vi "Scan Module.vi"(6 "Init":bool, 7 "Action":T1, 8 "Error In":errorcluster, 10 "Channel":u32(ring)=1 items=["A"=1, "B"=2, "A + B"=3, "C"=4, "A + C"=5, "A + B"=6, "D"=8, "A + D"=9, "B + D"=10, "C + D"=12, "A + B + C + D"=15], 11 "Mosaic Paramter":T2) -> (0 "Error Out":errorcluster, 1 "Current Position":cluster{"X":dbl, "Y":dbl}, 2 "Current State":T1, 3 "Finished?":bool)   [LabVIEW 2018]
uses:
  Controls/Go Scan Actions.ctl
  Controls/FGV Actions.ctl
  Hardware Mfg/Thorlabs Translation Stages/Controls/Motion Translation Module Control.ctl
  Hardware Mfg/Thorlabs Translation Stages/Controls/Translation Stage Cluster.ctl
  Controls/Translation Stage Types.ctl
  Controls/Set Get Controls.ctl
panel:
  out "Waveform Chart":dbl(graph)
  in  "No Slice?":bool
  out "XY Graph":cluster{"X":dbl, "Y":dbl}[](graph)
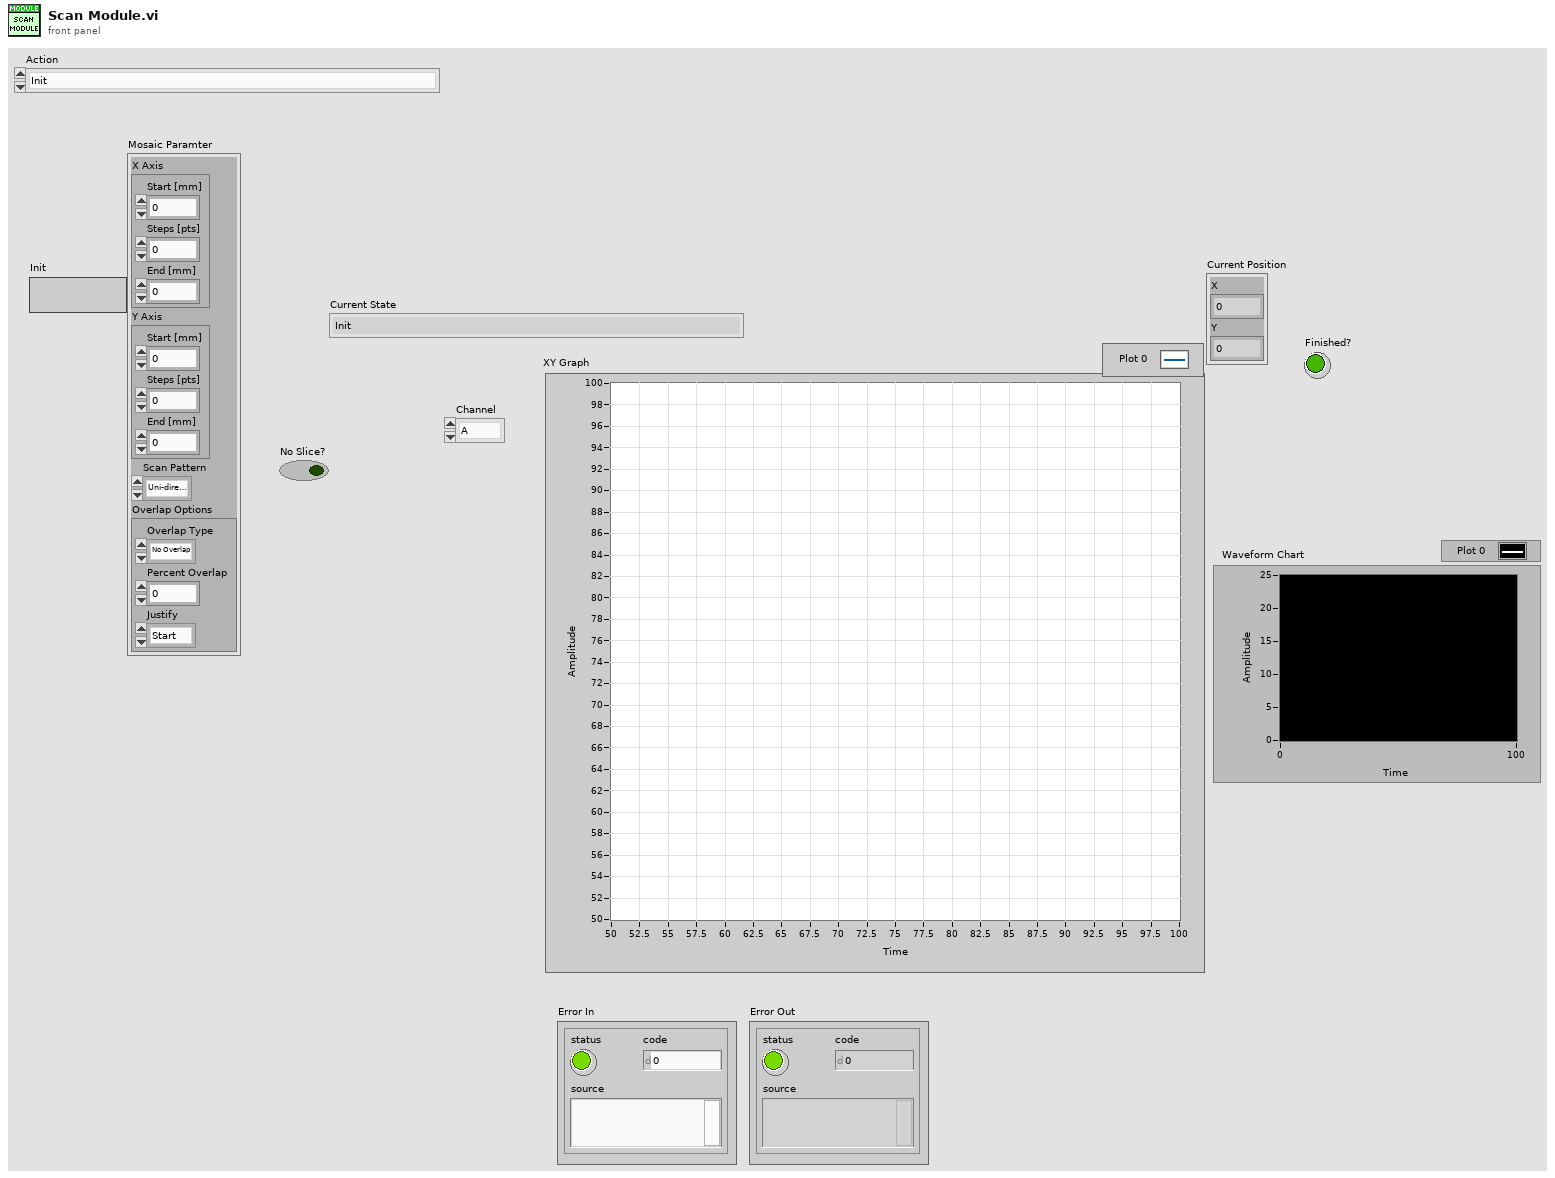
[diagram p1: front panel]
types:
  T1 = typedef "Go Scan Actions.ctl" = enum16{"Init", "Init Scan Head", "Init Table Stage", "Init Vibratome", "Generate Mosaic", "Go Image Home", "Go Mosaic", "Acquire Image", "Go Vibratome", "Slice", "Finished"}
  T2 = cluster{"X Axis":cluster{"Start [mm]":dbl, "Steps [pts]":u16, "End [mm]":dbl}, "Y Axis":cluster{"Start [mm]":dbl, "Steps [pts]":u16, "End [mm]":dbl}, "Scan Pattern":enum16{"Uni-directional", "Bi-Directional", "Spiral Out", "Spiral In"}, "Overlap Options":cluster{"Overlap Type":enum16{"No Overlap", "X Only", "Y Only", "X and Y"}, "Percent Overlap":u8, "Justify":enum16{"Start", "Center", "End"}}}
  T3 = typedef "FGV Actions.ctl" = enum16{"Init", "Set", "Get", "Clear"}
  T4 = typedef "Translation Stage Cluster.ctl" = cluster{"Position":dbl, "Is.Enabled?":bool, "Is.Connected?":bool, "Device SN":string, "AccelerationMaximum":dbl, "VelocityMaximum":dbl, "Acceleration":dbl, "Velocity":dbl, "waitTimeout (ms)":i32, "Model":T5, "Is.Homed?":bool}
  T5 = typedef "Translation Stage Types.ctl" = enum16{"None", "Thorlabs LTS", "Thorlabs MLJ"}
  T6 = typedef "Set Get Controls.ctl" = enum16{"Set", "Get"}
  T7 = typedef "Motion Translation Module Control.ctl" = enum16{"Init", "Home", "Status", "Velocity/Accel", "Position", "Jog", "Stop", "Uninit", "Enable", "Disable"}
  T8 = typedef "ScanType.ctl" = enum16{"Single Frame", "Continuous Frame", "ROI Line", "Vibratome", "Mosaic", "Mosaic + Slice"}
  T9 = cluster{"Start [mm]":dbl, "Steps [pts]":u16, "End [mm]":dbl}
  T10 = cluster{"Overlap Type":enum16{"No Overlap", "X Only", "Y Only", "X and Y"}, "Percent Overlap":u8, "Justify":enum16{"Start", "Center", "End"}}
  T11 = enum16{"Uni-directional", "Bi-Directional", "Spiral Out", "Spiral In"}
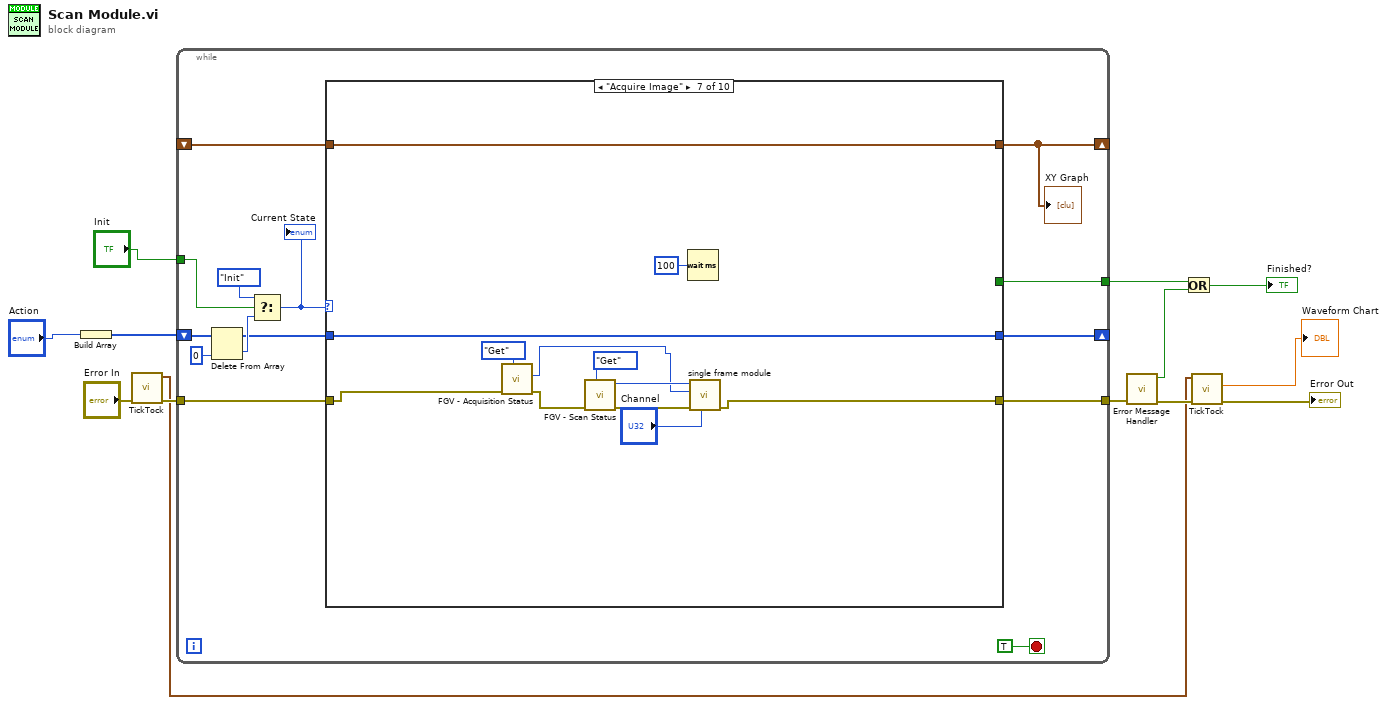
[diagram p0: block diagram]
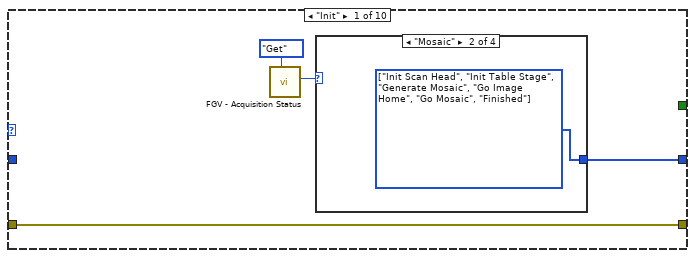
[diagram p2: hidden frame]
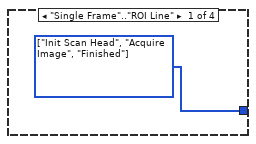
[diagram p3: hidden frame]
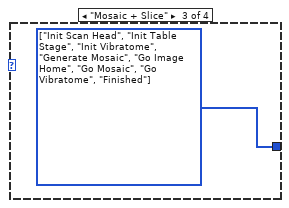
[diagram p4: hidden frame]
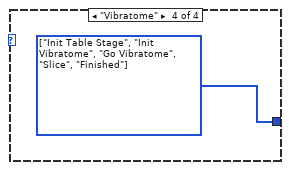
[diagram p5: hidden frame]
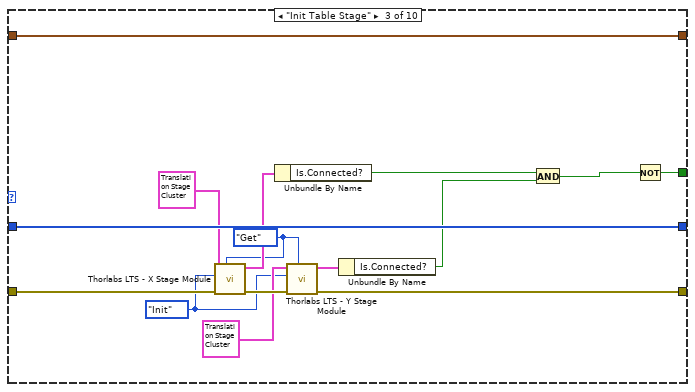
[diagram p7: hidden frame]
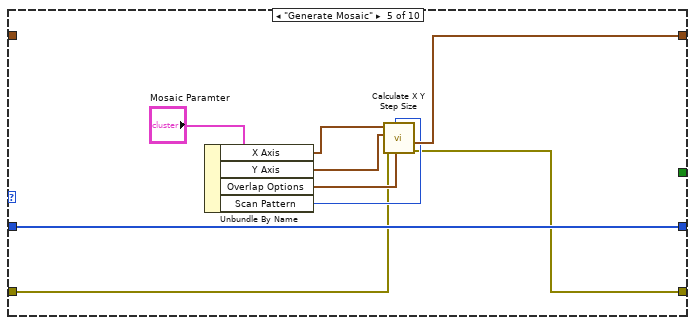
[diagram p9: hidden frame]
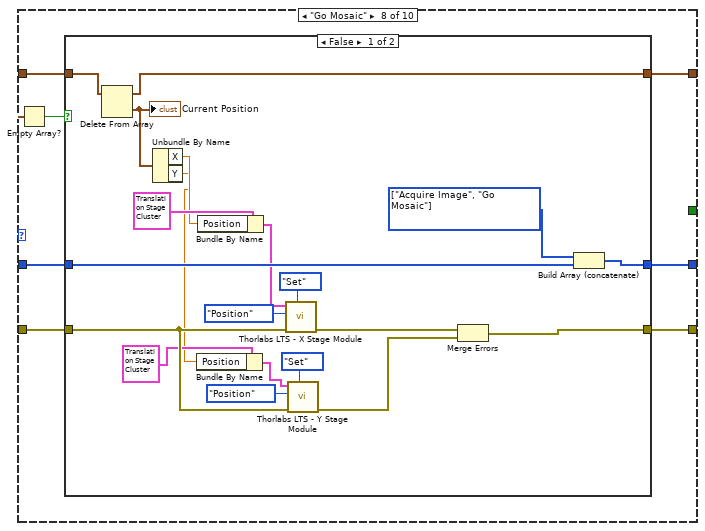
[diagram p11: hidden frame]
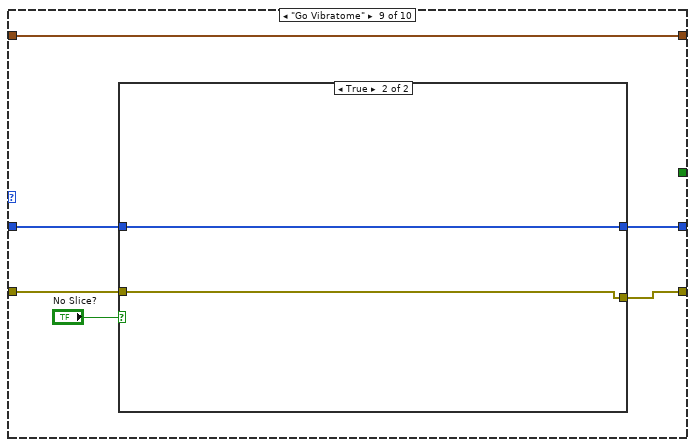
[diagram p13: hidden frame]
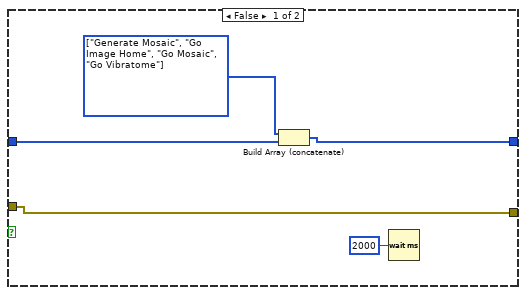
[diagram p14: hidden frame]
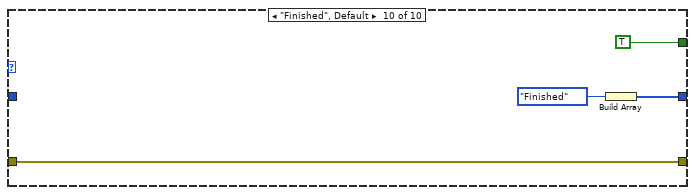
[diagram p15: hidden frame]
diagram:
  n1 = Build Array("Action") -> (w1:T1[])
  n2 = call "TickTock.vi"("Error In"="Error In") -> ("Error Out"=w6:errorcluster, "Current Time (Out)"=w4:timestamp)  [unwired: 8 in, 1 out]
  n3 = while {
    shift-right: [w23] -> _
    shift-left: w1 -> [w22]
    tunnel: "Init" -> [w25]
    shift-right: [w18] -> _
    shift-left: _ -> [w19]
    tunnel: [w17] -> w12
    tunnel: w6 -> [w15]
    tunnel: [w14] -> w11
    stop <- TRUE stop-if-true
    n4 = Delete From Array(array=w22, index=0) -> (deleted portion=w21:T1, array with subset deleted=w20:T1[])  [unwired: 1 in]
    n5 = Select(t=Go_Scan_Actions."Init", s=w25, f=w21) -> (s? t:f=w24:T1)
    "Current State" <- w24
    n6 = case shown="\"Acquire Image\"" w24 {
      tunnel: [w28 w37 w52 w55 w65 w67 w79 w83 w113 w126] -> w23
      tunnel: w20 -> [_ w37 w52 w55 w65 w67 w79 w84 w114 _]
      tunnel: [_ w38 w53 w56 w64 w68 w80 w87 w116 _] -> w18
      tunnel: w19 -> [_ w38 w53 w56 _ w68 w80 w86 w116 _]
      tunnel: [_ _ w47 _ _ _ _ _ _ TRUE] -> w17
      tunnel: w15 -> [w29 w36 w51 w54 w58 w66 w71 w82 w112 w124]
      tunnel: [w29 w36 w45 w54 w57 w66 w73 w81 w111 w124] -> w14
      frame "Init" {
        n7 = call "FGV - Acquisition Status.vi"("Actions"=FGV_Actions."Get") -> ("Scan Type [Out]"=w30:T8)  [unwired: 8 in, 2 out]
        n8 = case shown="\"Mosaic\"" w30 {
          tunnel: [w32 w33 w34 w35] -> w28
          frame "Single Frame".."ROI Line" {
            w32 = T1[] [enum."Init Scan Head", enum."Acquire Image", enum."Finished"] items=["Init", "Init Scan Head", "Init Table Stage", "Init Vibratome", "Generate Mosaic", "Go Image Home", "Go Mosaic", "Acquire Image", "Go Vibratome", "Slice", "Finished"]
          }
          frame "Mosaic" {
            w33 = T1[] [enum."Init Scan Head", enum."Init Table Stage", enum."Generate Mosaic", enum."Go Image Home", enum."Go Mosaic", enum."Finished"] items=["Init", "Init Scan Head", "Init Table Stage", "Init Vibratome", "Generate Mosaic", "Go Image Home", "Go Mosaic", "Acquire Image", "Go Vibratome", "Slice", "Finished"]
          }
          frame "Mosaic + Slice" {
            w34 = T1[] [enum."Init Scan Head", enum."Init Table Stage", enum."Init Vibratome", enum."Generate Mosaic", enum."Go Image Home", enum."Go Mosaic", enum."Go Vibratome", enum."Finished"] items=["Init", "Init Scan Head", "Init Table Stage", "Init Vibratome", "Generate Mosaic", "Go Image Home", "Go Mosaic", "Acquire Image", "Go Vibratome", "Slice", "Finished"]
          }
          frame "Vibratome" {
            w35 = T1[] [enum."Init Table Stage", enum."Init Vibratome", enum."Go Vibratome", enum."Slice", enum."Finished"] items=["Init", "Init Scan Head", "Init Table Stage", "Init Vibratome", "Generate Mosaic", "Go Image Home", "Go Mosaic", "Acquire Image", "Go Vibratome", "Slice", "Finished"]
          }
        }
      }
      frame "Init Scan Head" {
      }
      frame "Init Table Stage" {
        w39 = Set_Get_Controls."Get" ("Set/Get")
        w43 = Motion_Translation_Module_Control."Init" ("Action")
        n9 = call "Thorlabs LTS - X Stage Module.vi"("Set/Get"=w39, "Error In"=w51, "Action"=w43, "Cluster In"=T4 {"Position"=0.0, "Is.Enabled?"=TRUE, "Is.Connected?"=FALSE, "Device SN"="45876060", "AccelerationMaximum"=0.0, "VelocityMaximum"=0.0, "Acceleration"=0.0, "Velocity"=0.0, "waitTimeout (ms)"=10000, "Model"=enum."None", "Is.Homed?"=FALSE}) -> ("Error Out"=w50:errorcluster, "Cluster Out"=w49:T4)  [unwired: 6 in]
        n10 = Unbundle By Name(w49) -> ("Is.Connected?"=w48:bool)
        n11 = call "Thorlabs LTS - Y Stage Module.vi"("Set/Get"=w39, "Error In"=w50, "Action"=w43, "Cluster In"=T4 {"Position"=0.0, "Is.Enabled?"=TRUE, "Is.Connected?"=FALSE, "Device SN"="45876539", "AccelerationMaximum"=0.0, "VelocityMaximum"=0.0, "Acceleration"=0.0, "Velocity"=0.0, "waitTimeout (ms)"=10000, "Model"=enum."None", "Is.Homed?"=FALSE}) -> ("Error Out"=w45:errorcluster, "Cluster Out"=w42:T4)  [unwired: 6 in]
        n12 = Unbundle By Name(w42) -> ("Is.Connected?"=w40:bool)
        n13 = And(x=w48, y=w40) -> (x .and. y?=w41:bool)
        n14 = Not(x=w41) -> (.not. x?=w47:bool)
      }
      frame "Init Vibratome" {
      }
      frame "Generate Mosaic" {
        n15 = Unbundle By Name("Mosaic Paramter") -> ("X Axis"=w62:T9, "Y Axis"=w61:T9, "Overlap Options"=w60:T10, "Scan Pattern"=w59:T11)
        n16 = call "Calculate X Y Step Size.vi"("Overlap Options"=w60, "Scan Pattern"=w59, "Error In"=w58, "Y Axis"=w61, "X Axis"=w62) -> ("Error Out"=w57:errorcluster, "Array"=w64:cluster{"X":dbl, "Y":dbl}[])  [unwired: 3 in, 2 out]
      }
      frame "Go Image Home" {
      }
      frame "Acquire Image" {
        n17 = call "FGV - Acquisition Status.vi"("Actions"=FGV_Actions."Get", "Error In"=w71) -> ("Error Out"=w70:errorcluster, "Scan Type [Out]"=w69:T8)  [unwired: 7 in, 1 out]
        n18 = call "FGV - Scan Status.vi"("Actions"=FGV_Actions."Get", "Error In"=w70) -> ("Error Out"=w76:errorcluster, "Scan Status out"=w75:enum16{"Start", "Continue Scan", "Finish Scan"})  [unwired: 7 in, 1 out]
        n19 = Wait (ms)(milliseconds to wait=u32 100) -> ()  [unwired: 1 out]
        n20 = call "single frame module.vi"("Channel"="Channel", "Error in"=w76, "Scan Type in"=w69, "Scan Status in"=w75) -> ("Error Out"=w73:errorcluster)  [unwired: 7 in]
      }
      frame "Go Mosaic" {
        n21 = Empty Array?(array=w86) -> (empty?=w85:bool)
        n22 = case shown="False" w85 {
          tunnel: [w107 w110] -> w87
          tunnel: w86 -> [w106 w110]
          tunnel: w84 -> [w105 w109]
          tunnel: [w103 w109] -> w83
          tunnel: w82 -> [w93 w108]
          tunnel: [w89 w108] -> w81
          frame False {
            w102 = T1[] [enum."Acquire Image", enum."Go Mosaic"] items=["Init", "Init Scan Head", "Init Table Stage", "Init Vibratome", "Generate Mosaic", "Go Image Home", "Go Mosaic", "Acquire Image", "Go Vibratome", "Slice", "Finished"]
            n23 = Delete From Array(array=w106) -> (deleted portion=w104:cluster{"X":dbl, "Y":dbl}, array with subset deleted=w107:cluster{"X":dbl, "Y":dbl}[])  [unwired: 2 in]
            "Current Position" <- w104
            n24 = Unbundle By Name(w104) -> ("X"=w97:dbl, "Y"=w91:dbl)
            n25 = Bundle By Name(cluster=T4 {"Position"=0.0, "Is.Enabled?"=FALSE, "Is.Connected?"=FALSE, "Device SN"="45876539", "AccelerationMaximum"=0.0, "VelocityMaximum"=0.0, "Acceleration"=0.0, "Velocity"=0.0, "waitTimeout (ms)"=10000, "Model"=enum."None", "Is.Homed?"=FALSE} ("Cluster In"), "Position"=w91) -> (w90:T4)
            n26 = Bundle By Name(cluster=T4 {"Position"=0.0, "Is.Enabled?"=FALSE, "Is.Connected?"=FALSE, "Device SN"="45876539", "AccelerationMaximum"=0.0, "VelocityMaximum"=0.0, "Acceleration"=0.0, "Velocity"=0.0, "waitTimeout (ms)"=10000, "Model"=enum."None", "Is.Homed?"=FALSE} ("Cluster In"), "Position"=w97) -> (w96:T4)
            n27 = call "Thorlabs LTS - X Stage Module.vi"("Set/Get"=Set_Get_Controls."Set", "Error In"=w93, "Action"=Motion_Translation_Module_Control."Position", "Cluster In"=w96) -> ("Error Out"=w100:errorcluster)  [unwired: 6 in, 1 out]
            n28 = call "Thorlabs LTS - Y Stage Module.vi"("Set/Get"=Set_Get_Controls."Set", "Error In"=w93, "Action"=Motion_Translation_Module_Control."Position", "Cluster In"=w90) -> ("Error Out"=w88:errorcluster)  [unwired: 6 in, 1 out]
            n29 = Merge Errors(w100, w88) -> (w89:errorcluster)
            n30 = Build Array (concatenate)(w102, w105) -> (w103:T1[])
          }
          frame True {
          }
        }
      }
      frame "Go Vibratome" {
        n31 = case shown="True" "No Slice?" {
          tunnel: w114 -> [w121 w123]
          tunnel: [w120 w123] -> w113
          tunnel: w112 -> [w117 w122]
          tunnel: [w117 w122] -> w111
          frame False {
            w119 = T1[] [enum."Generate Mosaic", enum."Go Image Home", enum."Go Mosaic", enum."Go Vibratome"] items=["Init", "Init Scan Head", "Init Table Stage", "Init Vibratome", "Generate Mosaic", "Go Image Home", "Go Mosaic", "Acquire Image", "Go Vibratome", "Slice", "Finished"]
            n32 = Build Array (concatenate)(w119, w121) -> (w120:T1[])
            n33 = Wait (ms)(milliseconds to wait=u32 2000) -> ()  [unwired: 1 out]
          }
          frame True {
          }
        }
      }
      frame "Finished", Default {
        n34 = Build Array(Go_Scan_Actions."Finished") -> (w126:T1[])
      }
    }
    "XY Graph" <- w18
  }
  n35 = call "Error Message Handler.vi"("Error In"=w11) -> ("Error Out"=w10:errorcluster, "T button?"=w8:bool)  [unwired: 9 in]
  n36 = Or(x=w12, y=w8) -> (x .or. y?=→"Finished?":bool)
  n37 = call "TickTock.vi"("Error In"=w10, "Current Time (In)"=w4) -> ("Error Out"=→"Error Out":errorcluster, "dt"=→"Waveform Chart":dbl)  [unwired: 7 in, 1 out]
